vi "ni579x Get FAM CLIP Error.vi"(0 "Register Bus":refnum<class "ni579x Register Bus v1 Host.lvclass">=refnum, 11 "Error In":errorcluster) -> (4 "Register Bus (out)":refnum<class "ni579x Register Bus v1 Host.lvclass">, 15 "Error Out":errorcluster)   [LabVIEW 2013]
uses:
  <instrlib>/ni579x/Register Bus/v1/Host/ni579x Register Bus v1 Host.lvclass
  <instrlib>/ni579x/Config/v1/Shared/Types/ni579x Required FPGA Interface Reference.ctl
  <vilib>/rvi/interface/common/niFpgaWaitOnOcc.vi
  <vilib>/Utility/error.llb/Error Cluster From Error Code.vi
  <vilib>/rvi/errors/niLvFpgaAdjustHostInterfaceError.vi
  <vilib>/rvi/interface/nirviReadWriteControl/nirviReadWriteControl.xnode
  NiFpgaLv.dll
  <vilib>/rvi/interface/Simulation/niFpgaSimulationCallBeginRW.vi
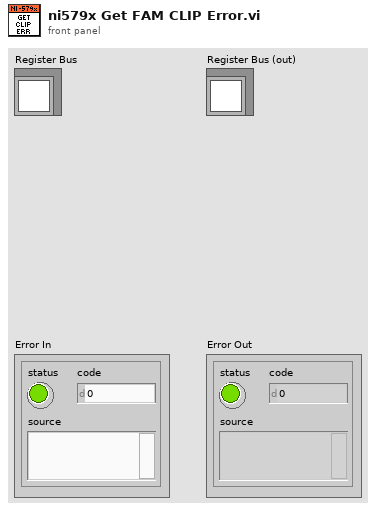
[diagram p1: front panel]
types:
  T1 = typedef "ni579x Required FPGA Interface Reference.ctl" = refnum<k20>
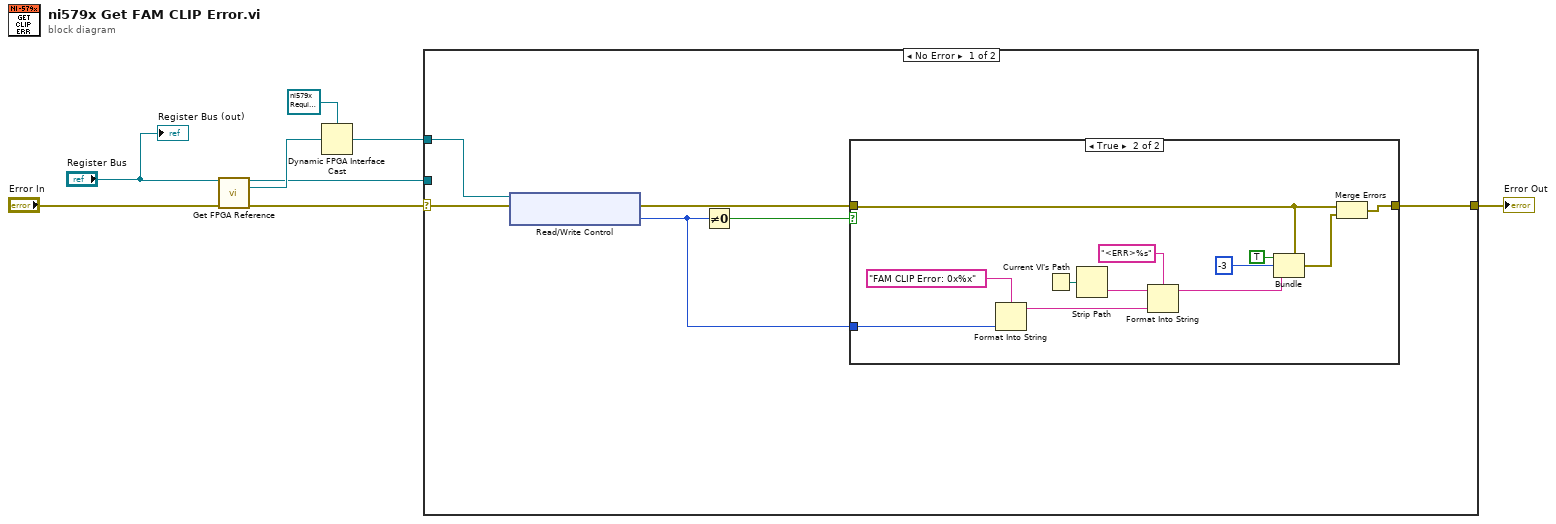
[diagram p0: block diagram]
diagram:
  n1 = call <instrlib>:"Get FPGA Reference.vi"("session in"="Register Bus", "error in"="Error In") -> ("session out"=w3:refnum<class "ni579x Register Bus v1 Host.lvclass">, "fpga ref"=w7:refnum<k20>, "error out"=w4:errorcluster)  [unwired: 11 in]
  n2 = Dynamic FPGA Interface Cast(Session In=T1 refnum ("Type"), Type=w7) -> (Session Out=w2:T1)
  n3 = case shown="No Error" w4 {
    selector: w4 -> [w10 w28]
    tunnel: [w11 w28] -> w8
    tunnel: w3 -> [_ _]
    tunnel: w2 -> [w14 _]
    frame No Error {
      n4 = xnode "Read/Write Control"("FPGA VI Reference In"=w14, "error in"=w10) -> ("error out"=w13:errorcluster, "IO Module\\User Error"=w12:u8)  [unwired: 1 out]
      n5 = Not Equal To 0?(x=w12) -> (x != 0?=w9:bool)
      n6 = case shown="True" w9 {
        tunnel: w13 -> [w15 w19]
        tunnel: [w15 w16] -> w11
        tunnel: w12 -> [_ w17]
        frame False {
        }
        frame True {
          n7 = Format Into String(format string="FAM CLIP Error: 0x%x" ("error message (\"\")"), w17) -> (resulting string=w18:string)  [unwired: 2 in, 1 out]
          n8 = Current VI's Path() -> (path=w25:path)
          n9 = Strip Path(path=w25) -> (name=w24:string)  [unwired: 1 out]
          n10 = Format Into String(format string="<ERR>%s", initial string=w24, w18) -> (resulting string=w23:string)  [unwired: 1 in, 1 out]
          n11 = Bundle(cluster=w19, "status"=TRUE, "code"=-3, "source"=w23) -> (w22:errorcluster)
          n12 = Merge Errors(w19, w22) -> (w16:errorcluster)
        }
      }
    }
    frame Error {
    }
  }
  "Error Out" <- w8
  "Register Bus (out)" <- "Register Bus"
